vi "alpha_0.1.vi"() -> ()   [LabVIEW 2018]
panel:
  out "Timer (s)":dbl
  out "P_RED":bool
  out "P_GREEN":bool
  in  "Emergency":bool
  in  "Waiter":dbl
  in  "?":bool
  out "RED":bool
  out "YELLOW":bool
  out "GREEN":bool
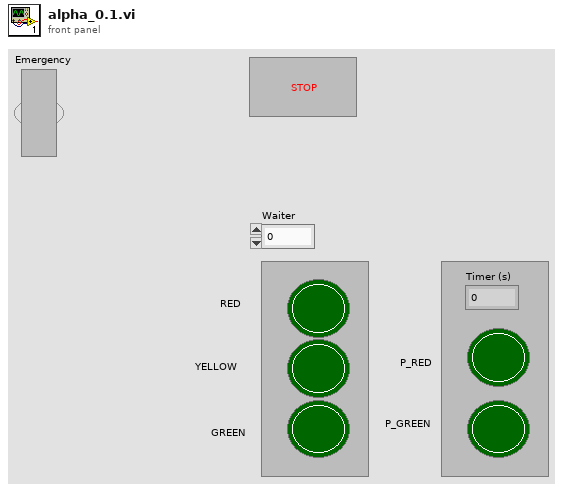
[diagram p1: front panel]
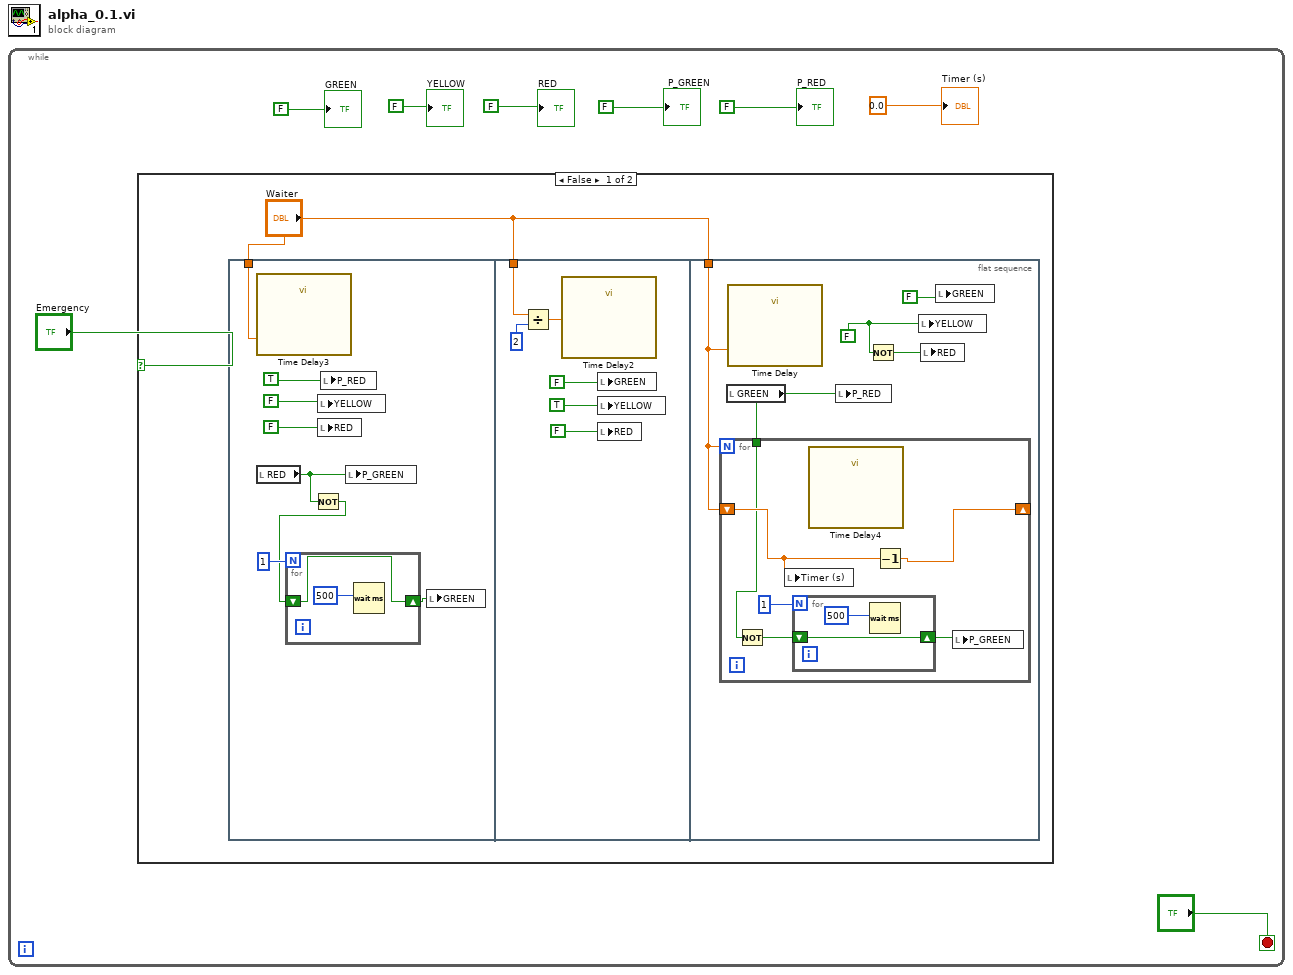
[diagram p0: block diagram]
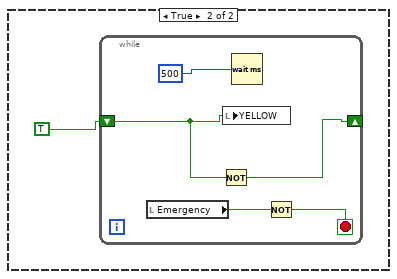
[diagram p2: hidden frame]
diagram:
  n1 = while {
    stop <- "?" stop-if-true
    n2 = case shown="False" "Emergency" {
      frame False {
        n3 = flat-sequence {
          tunnel: "Waiter" -> [w14]
          tunnel: "Waiter" -> [w22]
          tunnel: "Waiter" -> [w27]
          frame #0 {
            n4 = call "Time Delay3"("Delay Time (s)"=w14) -> ()  [unwired: 10 in, 1 out]
            n5 = local read "RED"() -> (w12:bool)
            n6 = Not(x=w12) -> (.not. x?=w11:bool)
            n7 = for {
              N: 1 -> [_]
              shift-right: [w18] -> w10
              shift-left: w11 -> [w18]
              n8 = Wait (ms)(milliseconds to wait=u32 500) -> ()  [unwired: 1 out]
            }
            n9 = local write "YELLOW"(FALSE) -> ()
            n10 = local write "RED"(FALSE) -> ()
            n11 = local write "P_RED"(TRUE) -> ()
            n12 = local write "P_GREEN"(w12) -> ()
            n13 = local write "GREEN"(w10) -> ()
          }
          frame #1 {
            n14 = Divide(x=w22, y=2) -> (x/y=w20:dbl)
            n15 = call "Time Delay2"("Delay Time (s)"=w20) -> ()  [unwired: 10 in, 1 out]
            n16 = local write "GREEN"(FALSE) -> ()
            n17 = local write "YELLOW"(TRUE) -> ()
            n18 = local write "RED"(FALSE) -> ()
          }
          frame #2 {
            w29 = FALSE
            n19 = local read "GREEN"() -> (w26:bool)
            n20 = for {
              N: w27 -> [_]
              shift-right: [w36] -> _
              shift-left: w27 -> [w35]
              tunnel: w26 -> [w31]
              n21 = Not(x=w31) -> (.not. x?=w33:bool)
              n22 = local write "Timer (s)"(w35) -> ()
              n23 = for {
                N: 1 -> [_]
                shift-right: [w38] -> w34
                shift-left: w33 -> [w38]
                n24 = Wait (ms)(milliseconds to wait=500) -> ()  [unwired: 1 out]
              }
              n25 = call "Time Delay4"() -> ()  [unwired: 11 in, 1 out]
              n26 = Decrement(x=w35) -> (x-1=w36:dbl)
              n27 = local write "P_GREEN"(w34) -> ()
            }
            n28 = call "Time Delay"("Delay Time (s)"=w27) -> ()  [unwired: 10 in, 1 out]
            n29 = local write "P_RED"(w26) -> ()
            n30 = Not(x=w29) -> (.not. x?=w28:bool)
            n31 = local write "YELLOW"(w29) -> ()
            n32 = local write "RED"(w28) -> ()
            n33 = local write "GREEN"(FALSE) -> ()
          }
        }
      }
      frame True {
        n34 = while {
          shift-right: [w43] -> _
          shift-left: TRUE -> [w44]
          stop <- w40 stop-if-true
          n35 = local read "Emergency"() -> (w41:bool)
          n36 = Not(x=w44) -> (.not. x?=w43:bool)
          n37 = local write "YELLOW"(w44) -> ()
          n38 = Wait (ms)(milliseconds to wait=500) -> ()  [unwired: 1 out]
          n39 = Not(x=w41) -> (.not. x?=w40:bool)
        }
      }
    }
    "GREEN" <- FALSE
    "YELLOW" <- FALSE
    "RED" <- FALSE
    "P_GREEN" <- FALSE
    "P_RED" <- FALSE
    "Timer (s)" <- 0.0
  }
